vi "Get Timing.vi"(8 "error in (no error)":errorcluster, 11 "RP Transceiver in":refnum<class "RP Transceiver.lvclass">) -> (0 "error out":errorcluster, 1 "dt":dbl, 2 "Total decimation":u32, 3 "RP Transceiver out":refnum<class "RP Transceiver.lvclass">, 4 "Logic clock rate":dbl=125000000.0)   [LabVIEW 2016, in "RP Transceiver.lvclass"]
uses:
  RP Transceiver.lvclass
  RP Transceiver.lvclass/RP Transceiver.ctl
  Read Total decimation.vi
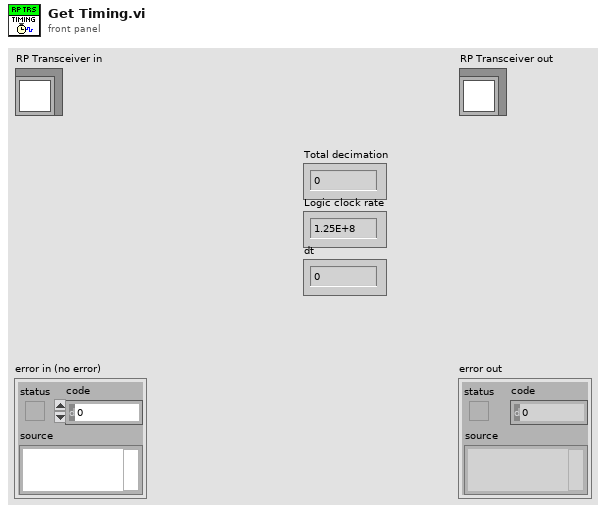
[diagram p1: front panel]
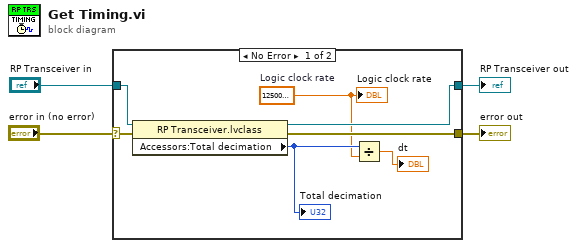
[diagram p0: block diagram]
diagram:
  n1 = case shown="No Error" "error in (no error)" {
    selector: "error in (no error)" -> [w11 w13]
    tunnel: [w10 w13] -> w3
    tunnel: [w8 w12] -> w1
    tunnel: "RP Transceiver in" -> [w9 w12]
    frame No Error {
      w6 = 125000000.0  # Logic clock rate
      n2 = property class="RP Transceiver.lvclass"(reference=w9, error in=w11) -> (reference out=w8:refnum<class "RP Transceiver.lvclass">, error out=w10:errorcluster, "Accessors:Total decimation"=w7:u32)
      "Total decimation" <- w7
      n3 = Divide(x=w7, y=w6) -> (x/y=→"dt":dbl)
      "Logic clock rate" <- w6
    }
    frame Error {
    }
  }
  "error out" <- w3
  "RP Transceiver out" <- w1
